vi "Measurement.vi"(7 "정지":bool, 8 "error in":errorcluster caption="에러 입력", 9 "Gyro Sensor":tag caption="물리적 채널", 11 "counter":tag caption="카운터") -> ()   [LabVIEW 2014]
uses:
  <vilib>/Analysis/baseanly.llb/Mean (DBL).vi
  <vilib>/DAQmx/create/channels.llb/DAQmx Create Channel (CI-Position-Linear Encoder).vi
  <vilib>/DAQmx/create/channels.llb/DAQmx Create Channel (AI-Voltage-Basic).vi
  <vilib>/DAQmx/configure/timing.llb/DAQmx Timing (Sample Clock).vi
  <vilib>/DAQmx/read.llb/DAQmx Read (Analog 1D DBL 1Chan NSamp).vi
  <vilib>/DAQmx/read.llb/DAQmx Read (Counter DBL 1Chan 1Samp).vi
  <vilib>/Analysis/NI_AALBase.lvlib
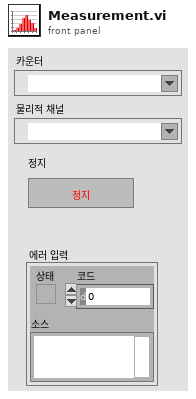
[diagram p1: front panel]
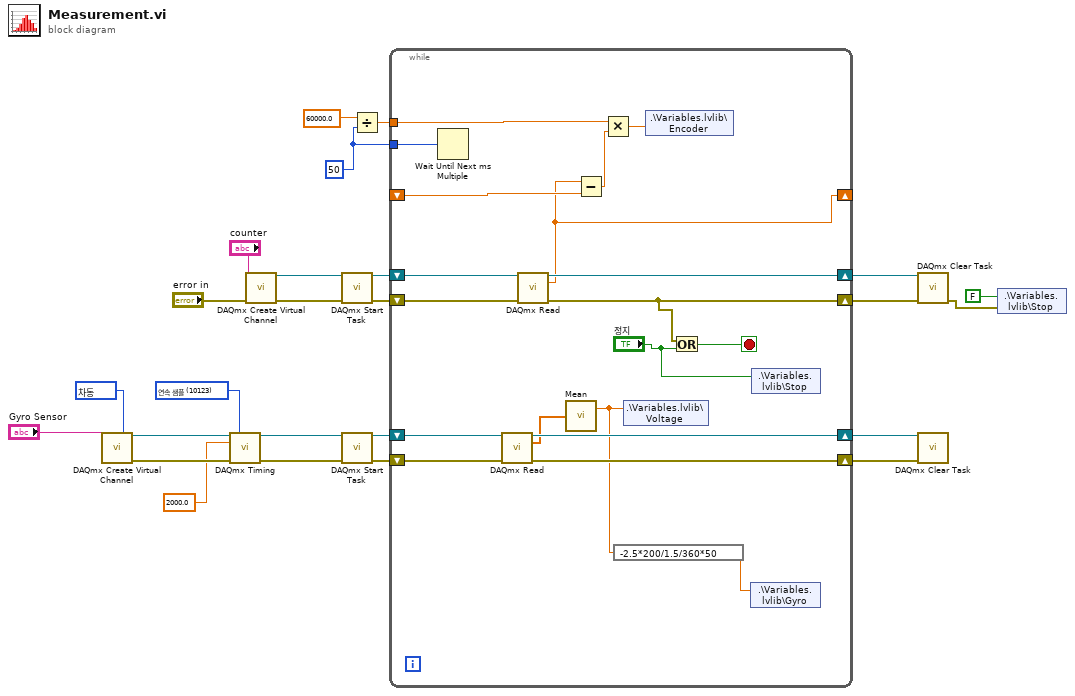
[diagram p0: block diagram]
diagram:
  w1 = 10123 items=["유한 샘플"=10178, "연속 샘플"=10123, "하드웨어 타이밍에 의한 단일 포인트"=12522] ("sample mode")
  w7 = 50
  w17 = 10106 items=["기본값"=-1, "RSE"=10083, "NRSE"=10078, "차동"=10106, "유사 차동"=12529] ("input terminal configuration")
  n1 = call-poly <vilib>:"DAQmx Create Virtual Channel.vi"("input terminal configuration"=w17, "physical channels"="Gyro Sensor") -> ("task out"=w15:refnum<k21>, "error out"=w14:errorcluster)  [unwired: 12 in]
  n2 = call-poly <vilib>:"DAQmx Timing.vi"("task/channels in"=w15, "sample mode"=w1, "rate"=2000.0, "error in"=w14) -> ("task out"=w13:refnum<k21>, "error out"=w12:errorcluster)  [unwired: 10 in]
  n3 = call-poly <vilib>:"DAQmx Create Virtual Channel.vi"("counter"="counter", "error in"="error in") -> ("task out"=w23:refnum<k21>, "error out"=w22:errorcluster)  [unwired: 12 in]
  n4 = call <vilib>:"DAQmx Start Task.vi"("task/channels in"=w23, "error in"=w22) -> ("task out"=w21:refnum<k21>, "error out"=w20:errorcluster)  [unwired: 12 in]
  n5 = call <vilib>:"DAQmx Start Task.vi"("task/channels in"=w13, "error in"=w12) -> ("task out"=w11:refnum<k21>, "error out"=w10:errorcluster)  [unwired: 12 in]
  n6 = Divide(x=60000.0, y=w7) -> (x/y=w5:dbl)
  n7 = while {
    shift-right: [w42] -> w19
    shift-left: w21 -> [w44]
    shift-right: [w31] -> w18
    shift-left: w20 -> [w43]
    shift-right: [w39] -> w9
    shift-left: w11 -> [w41]
    shift-right: [w38] -> w8
    shift-left: w10 -> [w40]
    tunnel: w7 -> [w37]
    tunnel: w5 -> [w36]
    shift-right: [w34] -> _
    shift-left: _ -> [w35]
    stop <- w30 stop-if-true
    n8 = Wait Until Next ms Multiple(millisecond multiple=w37) -> ()  [unwired: 1 out]
    n9 = call-poly <vilib>:"DAQmx Read.vi"("task/channels in"=w41, "error in"=w40) -> ("task out"=w39:refnum<k21>, "data"=w29:dbl[], "error out"=w38:errorcluster)  [unwired: 11 in]
    n10 = call-poly <vilib>:"DAQmx Read.vi"("task/channels in"=w44, "error in"=w43) -> ("task out"=w42:refnum<k21>, "data"=w34:dbl, "error out"=w31:errorcluster)  [unwired: 11 in]
    n11 = call-poly <vilib>:"Mean.vi"("X"=w29) -> ("mean"=w28:dbl)  [unwired: 1 out]
    n12 = Subtract(x=w34, y=w35) -> (x-y=w33:dbl)
    n13 = Multiply(x=w36, y=w33) -> (x*y=w32:dbl)
    n14 = expression code="-2.5*200/1.5/360*50"(w28) -> (w27:dbl)
    n15 = shared-variable ".\\Variables.lvlib\\Voltage"(w28) -> ()  [unwired: 1 in, 1 out]
    n16 = shared-variable ".\\Variables.lvlib\\Encoder"(w32) -> ()  [unwired: 1 in, 1 out]
    n17 = Or(x=w31, y="정지") -> (x .or. y?=w30:bool)
    n18 = shared-variable ".\\Variables.lvlib\\Gyro"(w27) -> ()  [unwired: 1 in, 1 out]
    n19 = shared-variable ".\\Variables.lvlib\\Stop"("정지") -> ()  [unwired: 1 in, 1 out]
  }
  n20 = call <vilib>:"DAQmx Clear Task.vi"("task in"=w19, "error in"=w18) -> ("error out"=w4:errorcluster)  [unwired: 13 in]
  n21 = call <vilib>:"DAQmx Clear Task.vi"("task in"=w9, "error in"=w8) -> ()  [unwired: 13 in, 1 out]
  n22 = shared-variable ".\\Variables.lvlib\\Stop"(FALSE ("Stop"), error in=w4) -> ()  [unwired: 1 out]
